vi "Common Array Elements.vi"(9 "Short Array":string[](array[string]), 11 "Source Array":string[](array[string])) -> (1 "Source-Short":string[](array[string]), 3 "Common Elements":string[](array[string]))   [LabVIEW 2020]
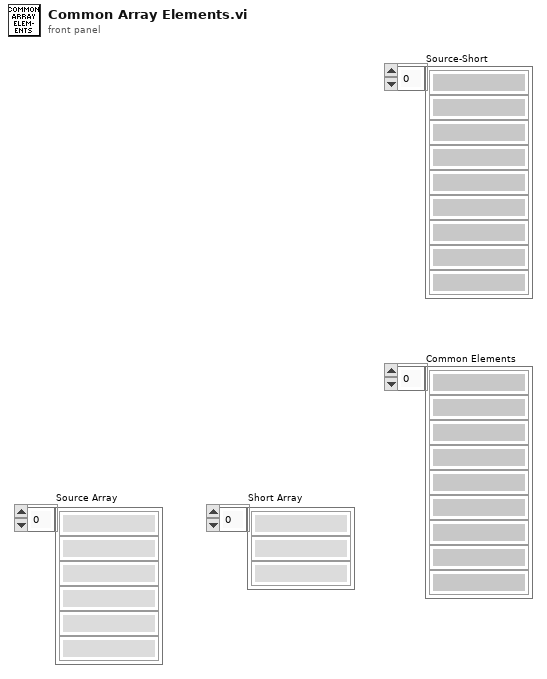
[diagram p1: front panel]
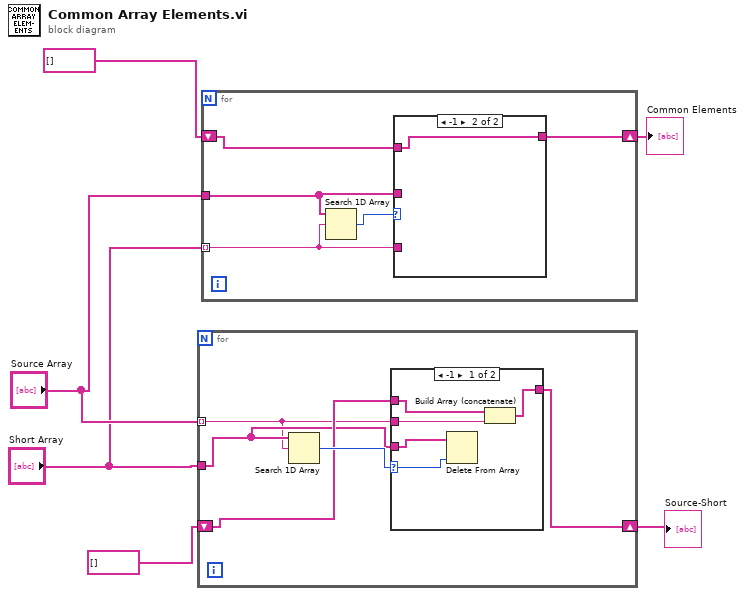
[diagram p0: block diagram]
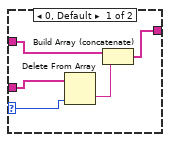
[diagram p3: hidden frame]
diagram:
  n1 = for {
    tunnel: "Source Array" -> [w7] mode=indexing
    tunnel: "Short Array" -> [w8]
    shift-right: [w9] -> w1
    shift-left: string[] [] -> [w10]
    n2 = Search 1D Array(1D array=w8, element=w7) -> (index of element=w11:i32)  [unwired: 1 in]
    n3 = case shown="-1" w11 {
      selector: w11 -> [w16 _]
      tunnel: w8 -> [w13 _]
      tunnel: w10 -> [w15 w17]
      tunnel: [w14 w17] -> w9
      tunnel: w7 -> [w12 _]
      frame -1 {
        n4 = Delete From Array(array=w13, index=w16) -> ()  [unwired: 1 in, 2 out]
        n5 = Build Array (concatenate)(w15, w12) -> (w14:string[])
      }
      frame 0, Default {
      }
    }
  }
  "Source-Short" <- w1
  n6 = for {
    tunnel: "Short Array" -> [w18] mode=indexing
    tunnel: "Source Array" -> [w22]
    shift-right: [w19] -> w6
    shift-left: string[] [] -> [w20]
    n7 = Search 1D Array(1D array=w22, element=w18) -> (index of element=w21:i32)  [unwired: 1 in]
    n8 = case shown="-1" w21 {
      selector: w21 -> [w27 _]
      tunnel: w22 -> [w23 _]
      tunnel: w20 -> [w26 w28]
      tunnel: [w25 w28] -> w19
      tunnel: w18 -> [_ _]
      frame 0, Default {
        n9 = Delete From Array(array=w23, index=w27) -> (deleted portion=w24:string)  [unwired: 1 in, 1 out]
        n10 = Build Array (concatenate)(w26, w24) -> (w25:string[])
      }
      frame -1 {
      }
    }
  }
  "Common Elements" <- w6
